vi "Read ADC.vi"() -> ()   [LabVIEW 2017]
uses:
  <vilib>/rvi/eio/common/nirviEmuTemplateMethod_errors.vi
  <vilib>/eio/EIONode/EIONode.xnode
panel:
  in  "ADC CS line":refnum<k21>="AI_CS1"
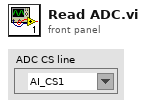
[diagram p1: front panel]
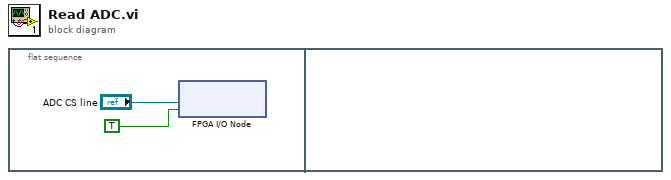
[diagram p0: block diagram]
diagram:
  n1 = flat-sequence {
    frame #0 {
      n2 = xnode "FPGA I/O Node"("I/O Item"=TRUE, "FPGA I/O In"="ADC CS line") -> ()  [unwired: 1 out]
    }
    frame #1 {
    }
  }
